vi "2182A and 2400 Combined Measuring V2.vi"() -> ()   [LabVIEW 2022 SP3]
uses:
  <vilib>/Analysis/baseanly.llb/Mean (DBL).vi
  <vilib>/Analysis/NI_AALBase.lvlib
  <instrlib>/Keithley 2182/Keithley 2182.lvlib
  Keithley 24XX Sweep and Acquire Measurements Folder/Keithley 24XX.lvlib
panel:
  in  "Resistance Measurement":T1(tab)
  in  "Measurement (1: Voltage Channel 1)":i32(ring)=1 items=["Voltage Channel 1"=1, "Voltage Channel 2"=2]
  in  "Source Mode  (0: Voltage)":u16(ring)=1 items=["Voltage", "Current"]
  in  "Compliance Level (0.1)":dbl=42.0
  in  "Current (µA)":dbl
  in  "2182A":T2={"Baud Rate"=9600, "Parity"=0, "Data Bits"=8, "Stop Bits"=10, "Flow Control"=0, "VISA resource name"="NanoVoltMeter"} {"Flow Control" items=["None", "XON/XOFF", "RTS/CTS", "XON/XOFF & RTS/CTS", "DTR/DSR", "XON/XOFF & DTR/DSR"]; "Stop Bits" items=["1.0"=10, "1.5"=15, "2.0"=20]; "Data Bits" items=["7"=7, "8"=8]; "Parity" items=["None", "Odd", "Even", "Mark", "Space"]; "Baud Rate" items=["300"=300, "600"=600, "1200"=1200, "2400"=2400, "4800"=4800, "9600"=9600, "19200"=19200]}
  in  "2400":T2={"Baud Rate"=9600, "Parity"=0, "Data Bits"=8, "Stop Bits"=10, "Flow Control"=0, "VISA resource name"="SourceMeter"} {"Flow Control" items=["None", "XON/XOFF", "RTS/CTS", "XON/XOFF & RTS/CTS", "DTR/DSR", "XON/XOFF & DTR/DSR"]; "Stop Bits" items=["1.0"=10, "1.5"=15, "2.0"=20]; "Data Bits" items=["7"=7, "8"=8]; "Parity" items=["None", "Odd", "Even", "Mark", "Space"]; "Baud Rate" items=["300"=300, "600"=600, "1200"=1200, "2400"=2400, "4800"=4800, "9600"=9600, "19200"=19200]}
  out "New file path 2":path
  in  "Folder to save file to":path
  in  "Number of experiments to run":i32=1
  in  "Buffer Size of 2400 and 2182 For Each Experiment":i32=3
  in  "Time To Wait for Buffer to Fill (ms)":u32=5000
  in  "Range Value (12)":dbl=12.0
  in  "Autorange (T: Enable)":bool=TRUE
  in  "Integration Rate (5)":dbl=5.0
  in  "Voltage Resolution (8)":i32=8
  out "Voltage Read By 2182 For Each Experiment":dbl[](array[numeric])
  out "Mean of Voltage Over All Experiments":dbl
  out "Mean of Current Over All Experiments":dbl
  out "Standard Deviation Voltage":dbl
  out "Standard Deviation Current":dbl
  out "Resistance Calculated For Each Experiment":dbl[](array[numeric])
  out "Mean of Resistance Over All Experiments":dbl
  out "Standard Deviation Resistance":dbl
  out "Current Supplied By 2400 For Each Experiment":dbl[](array[numeric])
  # "2182"
  # "2400"
  # "Basic"
  # "42V recomended"
  # "2182"
  # "2400"
  # "Ext"
  # "Needs to be longer as size of buffer increases"
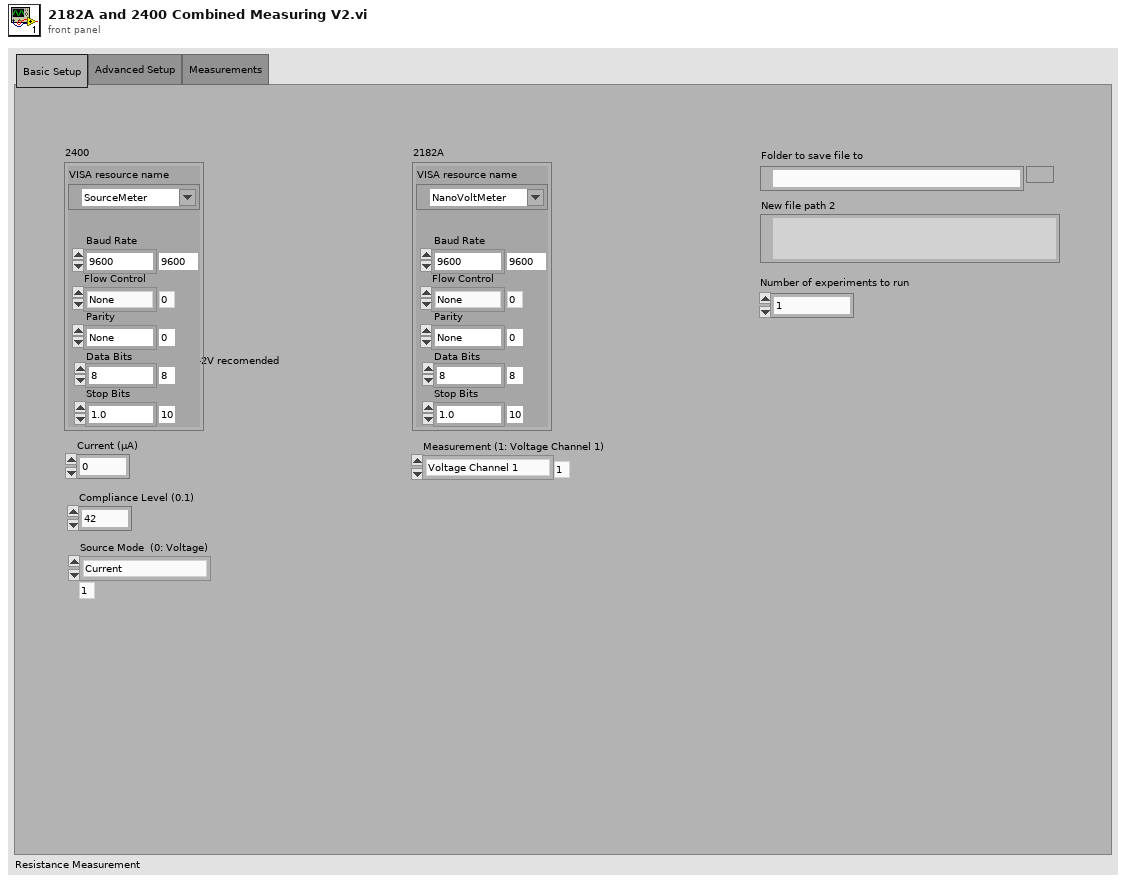
[diagram p1: front panel]
types:
  T1 = enum32{"Basic Setup", "Advanced Setup", "Measurements"}
  T2 = cluster{"Baud Rate":u32, "Parity":u16, "Data Bits":u16, "Stop Bits":u16, "Flow Control":u16, "VISA resource name":refnum<visa-resource-name>}
  T3 = enum16{"open", "replace", "create", "open or create", "replace or create", "replace or create with confirmation"}
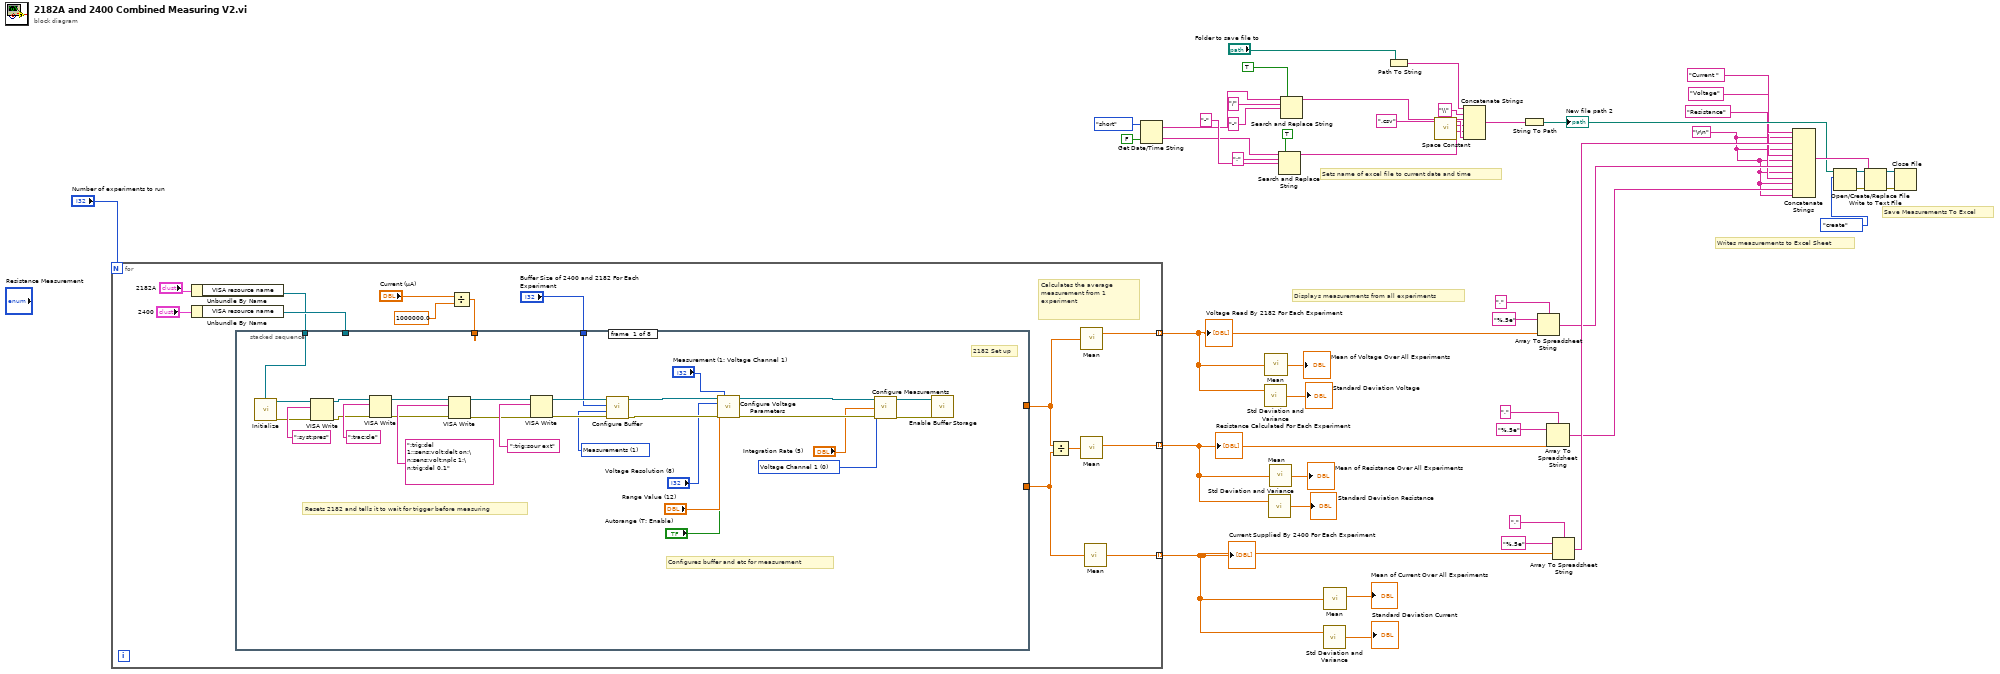
[diagram p0: block diagram]
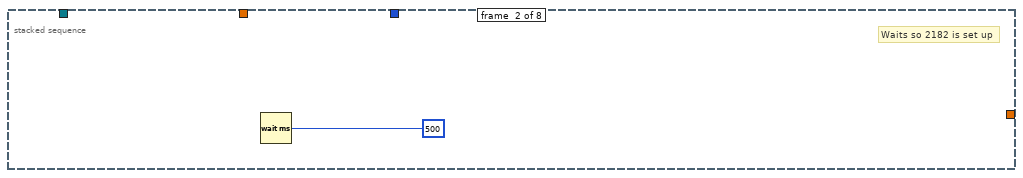
[diagram p2: hidden frame]
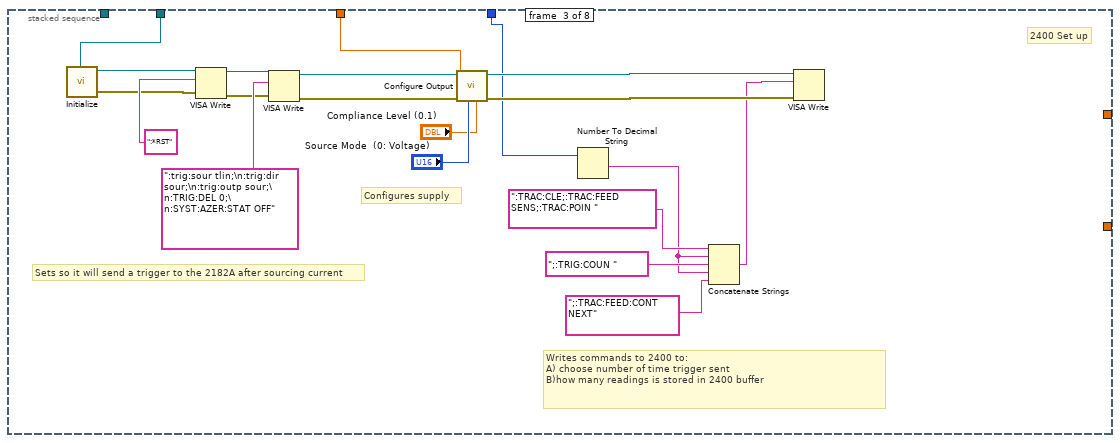
[diagram p3: hidden frame]
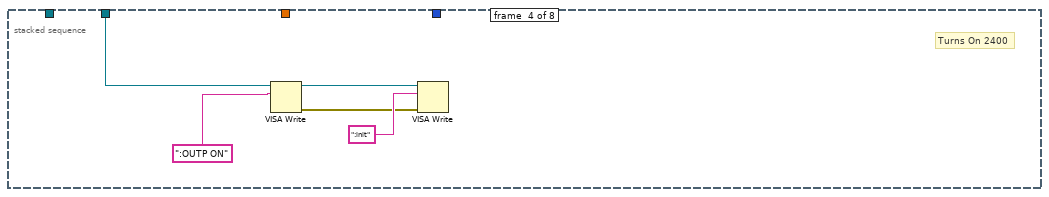
[diagram p4: hidden frame]
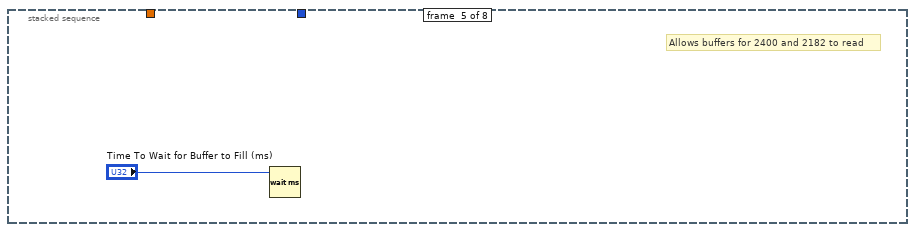
[diagram p5: hidden frame]
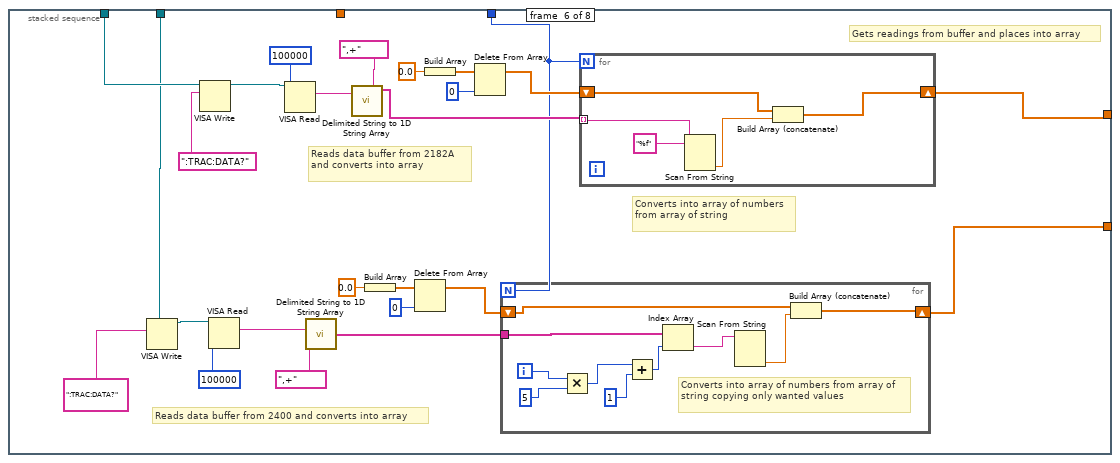
[diagram p6: hidden frame]
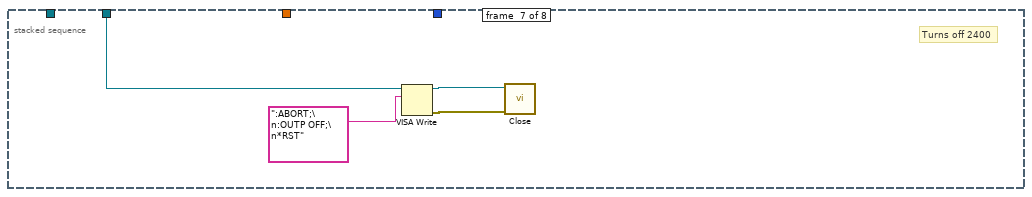
[diagram p7: hidden frame]
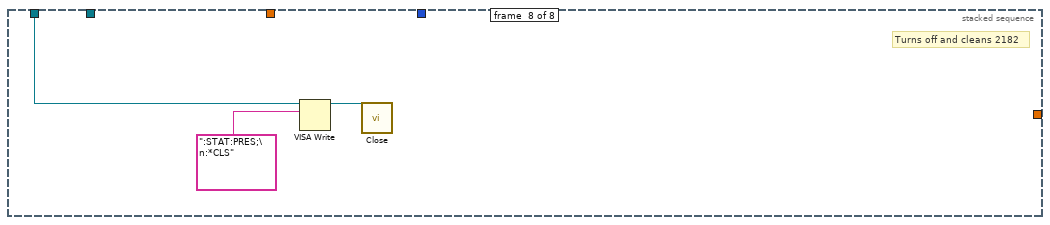
[diagram p8: hidden frame]
diagram:
  w6 = "\r\n"
  # "Displays measurements from all experiments"
  # "Writes measurements to Excel Sheet"
  # "Sets name of excel file to current date and time"
  # "Save Measurements To Excel"
  n1 = for {
    N: "Number of experiments to run" -> [_]
    tunnel: [w51] -> w1 mode=indexing
    tunnel: [w50] -> w3 mode=indexing
    tunnel: [w49] -> w2 mode=indexing
    # "Calculates the average measurement from 1 experiment"
    n2 = Unbundle By Name("2182A") -> ("VISA resource name"=w59:refnum<visa-resource-name>)
    n3 = Unbundle By Name("2400") -> ("VISA resource name"=w60:refnum<visa-resource-name>)
    n4 = Divide(x="Current (µA)", y=1000000.0) -> (x/y=w56:dbl)
    n5 = stacked-sequence {
      tunnel: w59 -> [w84 _ _ _ _ w137 _ w164]
      tunnel: w60 -> [_ _ w108 w117 _ w124 w159 _]
      tunnel: "Buffer Size of 2400 and 2182 For Each Experiment" -> [w68 _ w99 _ _ w120 _ _]
      tunnel: w56 -> [_ _ w102 _ _ _ _ _]
      tunnel: [_ _ _ _ _ w133 _ _] -> w54
      tunnel: [_ _ _ _ _ w119 _ _] -> w53
      frame #0 {
        w69 = 1 items=["None", "Measurements", "Math Calculation"] ("Buffer Source (0: None)")
        w81 = 0 items=["Voltage Channel 1", "Voltage Channel 2", "Temperature Channel 1", "Temperature Channel 2"] ("Measurement (0: Voltage Channel 1)")
        # "Configures buffer and etc for measurement"
        # "Resets 2182 and tells it to wait for trigger before measuring"
        # "2182 Set up"
        n6 = call <instrlib>:"Initialize.vi"("VISA resource name"=w84) -> ("error out"=w75:errorcluster, "VISA resource name out"=w83:refnum<visa-resource-name>)  [unwired: 9 in]
        n7 = VISA Write(VISA resource name=w83, write buffer=":syst:pres", error in (no error)=w75) -> (VISA resource name out=w85:refnum<visa-resource-name>, error out=w74:errorcluster)  [unwired: 1 out]
        n8 = VISA Write(VISA resource name=w85, write buffer=":trac:cle", error in (no error)=w74) -> (VISA resource name out=w87:refnum<visa-resource-name>, error out=w73:errorcluster)  [unwired: 1 out]
        n9 = VISA Write(VISA resource name=w87, write buffer=":trig:del 1;:sens:volt:delt on;\n:sens:volt:nplc 1;\n:trig:del 0.1", error in (no error)=w73) -> (VISA resource name out=w86:refnum<visa-resource-name>, error out=w72:errorcluster)  [unwired: 1 out]
        n10 = VISA Write(VISA resource name=w86, write buffer=":trig:sour ext", error in (no error)=w72) -> (VISA resource name out=w79:refnum<visa-resource-name>, error out=w77:errorcluster)  [unwired: 1 out]
        n11 = call <instrlib>:"Configure Buffer.vi"("error in (no error)"=w77, "Buffer Source (0: None)"=w69, "Buffer Size (2)"=w68, "VISA resource name"=w79) -> ("error out"=w76:errorcluster, "VISA resource name out"=w78:refnum<visa-resource-name>)  [unwired: 6 in]
        n12 = call <instrlib>:"Configure Voltage Parameters.vi"("VISA resource name"=w78, "Measurement (1: Voltage Channel 1)"="Measurement (1: Voltage Channel 1)", "Voltage Resolution (8)"="Voltage Resolution (8)", "Range Value (12)"="Range Value (12)", "Autorange (T: Enable)"="Autorange (T: Enable)", "error in (no error)"=w76) -> ("VISA resource name out"=w82:refnum<visa-resource-name>, "error out"=w71:errorcluster)  [unwired: 8 in]
        n13 = call <instrlib>:"Configure Measurements.vi"("VISA resource name"=w82, "Measurement (0: Voltage Channel 1)"=w81, "Integration Rate (5)"="Integration Rate (5)", "error in (no error)"=w71) -> ("VISA resource name out"=w80:refnum<visa-resource-name>, "error out"=w70:errorcluster)  [unwired: 10 in]
        n14 = call <instrlib>:"Enable Buffer Storage.vi"("error in (no error)"=w70, "VISA resource name"=w80) -> ()  [unwired: 8 in, 2 out]
      }
      frame #1 {
        # "Waits so 2182 is set up"
        n15 = Wait (ms)(milliseconds to wait=u32 500) -> ()  [unwired: 1 out]
      }
      frame #2 {
        # "Writes commands to 2400 to:\nA) choose number of time trigger sent \nB)how many readings is stored in 2400 buffer"
        # "Configures supply"
        # "Sets so it will send a trigger to the 2182A after sourcing current"
        # "2400 Set up"
        # "2400 Set Up"
        n16 = call <instrlib>:"Initialize.vi"("VISA resource name"=w108) -> ("error out"=w106:errorcluster, "VISA resource name out"=w107:refnum<visa-resource-name>)  [unwired: 9 in]
        n17 = VISA Write(VISA resource name=w107, write buffer=":*RST", error in (no error)=w106) -> (VISA resource name out=w112:refnum<visa-resource-name>, error out=w105:errorcluster)  [unwired: 1 out]
        n18 = VISA Write(VISA resource name=w112, write buffer=":trig:sour tlin;\n:trig:dir sour;\n:trig:outp sour;\n:TRIG:DEL 0;\n:SYST:AZER:STAT OFF", error in (no error)=w105) -> (VISA resource name out=w111:refnum<visa-resource-name>, error out=w104:errorcluster)  [unwired: 1 out]
        n19 = call "Configure Output.vi"("Source Mode  (0: Voltage)"="Source Mode  (0: Voltage)", "error in (no error)"=w104, "Compliance  Level (0.1)"="Compliance Level (0.1)", "Output Level (0)"=w102, "VISA resource name"=w111) -> ("error out"=w100:errorcluster, "VISA resource name out"=w101:refnum<visa-resource-name>)  [unwired: 5 in]
        n20 = Number To Decimal String(number=w99) -> (decimal integer string=w95:string)  [unwired: 1 in]
        n21 = Concatenate Strings(":TRAC:CLE;:TRAC:FEED SENS;:TRAC:POIN " ("write buffer"), w95, ";:TRIG:COUN " ("write buffer"), w95, ";:TRAC:FEED:CONT NEXT" ("write buffer")) -> (w97:string)
        n22 = VISA Write(VISA resource name=w101, write buffer=w97, error in (no error)=w100) -> ()  [unwired: 3 out]
      }
      frame #3 {
        # "Turns On 2400"
        n23 = VISA Write(VISA resource name=w117, write buffer=":OUTP ON") -> (VISA resource name out=w116:refnum<visa-resource-name>, error out=w113:errorcluster)  [unwired: 1 in, 1 out]
        n24 = VISA Write(VISA resource name=w116, write buffer=":init", error in (no error)=w113) -> ()  [unwired: 3 out]
      }
      frame #4 {
        # "Allows buffers for 2400 and 2182 to read"
        n25 = Wait (ms)(milliseconds to wait="Time To Wait for Buffer to Fill (ms)") -> ()  [unwired: 1 out]
      }
      frame #5 {
        # "Reads data buffer from 2400 and converts into array"
        # "Converts into array of numbers from array of string"
        # "Reads data buffer from 2182A and converts into array"
        # "Gets readings from buffer and places into array"
        n26 = VISA Write(VISA resource name=w124, write buffer=":TRAC:DATA?") -> (VISA resource name out=w131:refnum<visa-resource-name>)  [unwired: 1 in, 2 out]
        n27 = VISA Write(VISA resource name=w137, write buffer=":TRAC:DATA?") -> (VISA resource name out=w140:refnum<visa-resource-name>)  [unwired: 1 in, 2 out]
        n28 = VISA Read(VISA resource name=w131, byte count=u32 100000) -> (read buffer=w142:string)  [unwired: 1 in, 3 out]
        n29 = VISA Read(VISA resource name=w140, byte count=u32 100000) -> (read buffer=w135:string)  [unwired: 1 in, 3 out]
        n30 = call <vilib>:"Delimited String to 1D String Array.vi"("delimiter"=",+" ("delimiter (Tab)"), "delimited string"=w142) -> ("string array"=w122:string[])  [unwired: 9 in]
        n31 = call <vilib>:"Delimited String to 1D String Array.vi"("delimiter"=",+" ("delimiter (Tab)"), "delimited string"=w135) -> ("string array"=w134:string[])  [unwired: 9 in]
        n32 = Build Array(0.0 ("array")) -> (w126:dbl[])
        n33 = Delete From Array(array=w126, index=0) -> (array with subset deleted=w121:dbl[])  [unwired: 1 in, 1 out]
        n34 = Build Array(0.0 ("array")) -> (w129:dbl[])
        n35 = Delete From Array(array=w129, index=0) -> (array with subset deleted=w123:dbl[])  [unwired: 1 in, 1 out]
        n36 = for {
          N: w120 -> [_]
          tunnel: w122 -> [w153]
          shift-right: [w145] -> w119
          shift-left: w121 -> [w144]
          i -> [w152]
          # "Converts into array of numbers from array of string copying only wanted values"
          n37 = Multiply(x=w152, y=5) -> (x*y=w151:i32)
          n38 = Add(x=w151, y=1) -> (x+y=w148:i32)
          n39 = Index Array(array=w153, index=w148) -> (element=w147:string)
          n40 = Scan From String(input string=w147) -> (output 1=w146:dbl)  [unwired: 4 in, 3 out]
          n41 = Build Array (concatenate)(w144, w146) -> (w145:dbl[])
        }
        n42 = for {
          N: w120 -> [_]
          tunnel: w134 -> [w158] mode=indexing
          shift-right: [w155] -> w133
          shift-left: w123 -> [w154]
          n43 = Scan From String(format string="%f", input string=w158) -> (output 1=w156:dbl)  [unwired: 3 in, 3 out]
          n44 = Build Array (concatenate)(w154, w156) -> (w155:dbl[])
        }
      }
      frame #6 {
        # "Turns off 2400"
        n45 = VISA Write(VISA resource name=w159, write buffer=":ABORT;\n:OUTP OFF;\n*RST" ("data")) -> (VISA resource name out=w161:refnum<visa-resource-name>, error out=w160:errorcluster)  [unwired: 1 in, 1 out]
        n46 = call <instrlib>:"Close.vi"("error in (no error)"=w160, "VISA resource name"=w161) -> ()  [unwired: 9 in, 1 out]
      }
      frame #7 {
        # "Turns off and cleans 2182"
        n47 = VISA Write(VISA resource name=w164, write buffer=":STAT:PRES;\n:*CLS" ("data")) -> (VISA resource name out=w163:refnum<visa-resource-name>)  [unwired: 1 in, 2 out]
        n48 = call <instrlib>:"Close.vi"("VISA resource name"=w163) -> ()  [unwired: 10 in, 1 out]
      }
    }
    n49 = Divide(x=w54, y=w53) -> (x/y=w52:dbl[])
    n50 = call-poly <vilib>:"Mean.vi"("X"=w54) -> ("mean"=w51:dbl)  [unwired: 1 out]
    n51 = call-poly <vilib>:"Mean.vi"("X"=w52) -> ("mean"=w49:dbl)  [unwired: 1 out]
    n52 = call-poly <vilib>:"Mean.vi"("X"=w53) -> ("mean"=w50:dbl)  [unwired: 1 out]
  }
  "Voltage Read By 2182 For Each Experiment" <- w1
  "Resistance Calculated For Each Experiment" <- w2
  "Current Supplied By 2400 For Each Experiment" <- w3
  n53 = Get Date/Time String(date format (0)=enum16{"short", "long", "abbreviated"}."short", want seconds? (F)=FALSE) -> (date string=w30:string, time string=w35:string)  [unwired: 1 in]
  n54 = call <vilib>:"Std Deviation and Variance.vi"("X"=w1) -> ("standard deviation"=→"Standard Deviation Voltage":dbl)  [unwired: 1 in, 2 out]
  n55 = call-poly <vilib>:"Mean.vi"("X"=w1) -> ("mean"=→"Mean of Voltage Over All Experiments":dbl)  [unwired: 1 out]
  n56 = call <vilib>:"Std Deviation and Variance.vi"("X"=w2) -> ("standard deviation"=→"Standard Deviation Resistance":dbl)  [unwired: 1 in, 2 out]
  n57 = call-poly <vilib>:"Mean.vi"("X"=w2) -> ("mean"=→"Mean of Resistance Over All Experiments":dbl)  [unwired: 1 out]
  n58 = Search and Replace String(replace all?=TRUE ("replace all? (F)"), input string=w35, search string=":" ("replace string (\"\")"), replace string="-" ("replace string (\"\")")) -> (result string=w39:string)  [unwired: 4 in, 3 out]
  n59 = Search and Replace String(replace all?=TRUE, input string=w30, search string="/" ("replace string (\"\")"), replace string="-" ("replace string (\"\")")) -> (result string=w29:string)  [unwired: 4 in, 3 out]
  n60 = call <vilib>:"Std Deviation and Variance.vi"("X"=w3) -> ("standard deviation"=→"Standard Deviation Current":dbl)  [unwired: 1 in, 2 out]
  n61 = call-poly <vilib>:"Mean.vi"("X"=w3) -> ("mean"=→"Mean of Current Over All Experiments":dbl)  [unwired: 1 out]
  n62 = Path To String(path="Folder to save file to") -> (string=w43:string)
  n63 = call <vilib>:"Space Constant.vi"() -> ("String"=w38:string)
  n64 = Concatenate Strings "Concatenate Strings"(w43, "\\" ("string"), w29, w38, w39, ".csv" ("string")) -> (w41:string)
  n65 = String To Path(string=w41) -> (path=w17:path)
  "New file path 2" <- w17
  n66 = Array To Spreadsheet String(delimiter (Tab)=",", array=w1, 3:"%.5e") -> (spreadsheet string=w9:string)
  n67 = Array To Spreadsheet String(delimiter (Tab)=",", array=w2, 3:"%.5e") -> (spreadsheet string=w7:string)
  n68 = Array To Spreadsheet String(delimiter (Tab)=",", array=w3, 3:"%.5e") -> (spreadsheet string=w11:string)
  n69 = Concatenate Strings("Current ", w6, w11, w6, "Voltage", w6, w9, w6, "Resistance", w6, w7, w6) -> (w22:string)
  n70 = Open/Create/Replace File(file path (use dialog)=w17, operation (0:open)=T3."create") -> (refnum out=w25:refnum<file>, error out=w26:errorcluster)  [unwired: 4 in, 1 out]
  n71 = Write to Text File(file (use dialog)=w25, text=w22, error in=w26) -> (refnum out=w23:refnum<file>, error out=w24:errorcluster)  [unwired: 1 in, 1 out]
  n72 = Close File(refnum=w23, error in=w24) -> ()  [unwired: 2 out]
